vi "Actor Core.vi"(8 "error in (no error)":errorcluster, 11 "front_panel in":refnum<class "front_panel.lvclass">) -> (0 "error out":errorcluster, 3 "Actor out":refnum<class "Actor.lvclass">)   [LabVIEW 2015, in "front_panel.lvclass"]
doc: "(<B>Filename</B>: Actor Framework.lvlib:Actor.lvclass:Actor Core.vi)\n\nReceives messages to the actor, reacts to them, and initiates any error handling that may shut the actor down.\n\nDescendant classes may override this VI to append parallel tasks for the actor to complete while it handles messages. Overrides use the Call Parent Method node."
uses:
  front_panel.lvclass
  <vilib>/ActorFramework/Actor/Actor.lvclass
  stage_types.ctl
  experiment_types.ctl
  detector_types.ctl
  gui_subpanel_references.ctl
  ui_plot_references.ctl
  ui_elements.ctl
  front_panel.lvclass/front_panel.ctl
  panel_class/panel.lvclass/panel.ctl
  <vilib>/ActorFramework/Actor/Actor.lvclass/Actor.ctl
  <vilib>/ActorFramework/Message Enqueuer/Message Enqueuer.lvclass/Message Enqueuer.ctl
  front_panel Messages/replace_subpanel Msg/replace_subpanel Msg.lvclass/replace_subpanel Msg.ctl
  map_data.ctl
  <vilib>/Utility/miscctls.llb/LVOffsetAndMultiplierTypeDef.ctl
  <vilib>/ActorFramework/Message Enqueuer/Init from Existing Queue.vi
  <vilib>/ActorFramework/Message Enqueuer/Enqueue.vi
  <vilib>/ActorFramework/Message Priority Queue/Priority Enqueue.vi
  <vilib>/ActorFramework/Message Enqueuer/Message Enqueuer.lvclass
  <vilib>/ActorFramework/Stop Msg/Stop Msg.lvclass
  front_panel Messages/replace_subpanel Msg/replace_subpanel Msg.lvclass
  panel_class/panel.lvclass
panel:
  in  "stage1":T1
  in  "stage2":T1
  in  "experiment":T2
  in  "2.":T3
  in  "detector":T3
  in  "plots":T4(tab)
  in  "ch_4_color 2":u32(colorbox)=11141375 caption="6"
  in  "ch_3_color 2":u32(colorbox)=16768322 caption="5"
  out "Y Cursor":dbl
  out "X Cursor":dbl
  in  "ch_4_color":u32(colorbox)=3381759 caption="4"
  in  "ch_3_color":u32(colorbox)=6618880 caption="3"
  in  "ch_2_color":u32(colorbox)=16711680 caption="2"
  in  "ch_1_color":u32(colorbox)=13816530 caption="1"
  out "chart":cluster{dbl, dbl, dbl, dbl, dbl, dbl, dbl, dbl}(graph)
  out "graph":dbl[](graph)
  in  "load _map":bool
  in  "clear_maps":bool
  out "current":i32
  out "maps stored":i32
  in  "map_forward":bool
  in  "map_back":bool
  in  "keep_map":bool
  out "Y Cursor":dbl
  out "X Cursor":dbl
  out "map":dbl[][](graph)
  out "XY Graph":cluster{dbl[], dbl[]}[](graph)
  out "ch4":dbl
  out "ch3":dbl
  out "ch2":dbl
  out "ch1":dbl
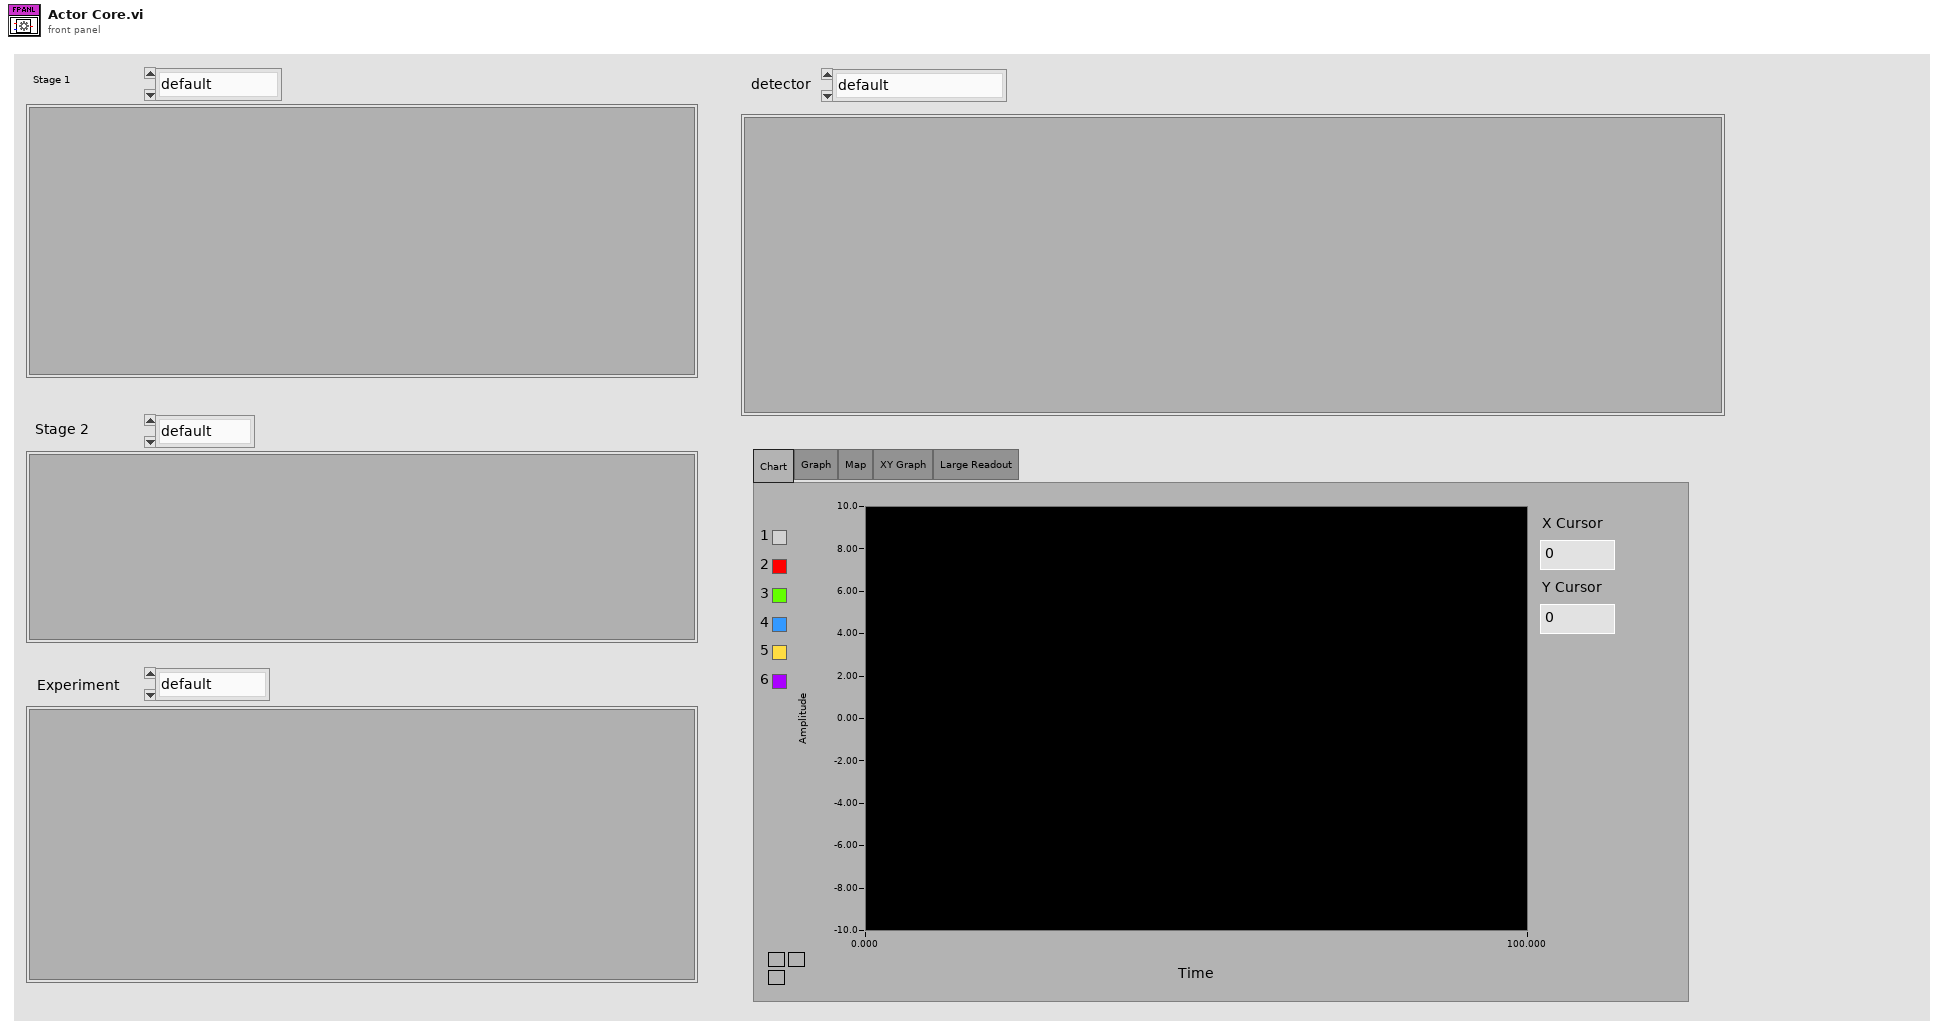
[diagram p1: front panel]
types:
  T1 = typedef "stage_types.ctl" = enum16{"default", "Newport XPS", "Aerotech Ensemble", "Galvos", "Throlabs Kinesis", "MCL XYZ Piezo"}
  T2 = typedef "experiment_types.ctl" = enum16{"default", "PCFS", "Scan", "2D Galvo Scan"}
  T3 = typedef "detector_types.ctl" = enum16{"default", "Hydraharp", "Picoharp", "Lightfield"}
  T4 = enum32{"Chart", "Graph", "Map", "XY Graph", "Large Readout"}
  T5 = typedef "ui_elements.ctl" = cluster{"map_xcursor":refnum<vi>, "map_ycursor":refnum<vi>}
  T6 = typedef "ui_plot_references.ctl" = cluster{"plots":refnum<vi>, "chart":refnum<vi>, "graph":refnum<vi>, "map":refnum<vi>, "XY Graph":refnum<vi>}
  T7 = typedef "gui_subpanel_references.ctl" = cluster{"Stage 1":refnum<vi>, "Stage 2":refnum<vi>, "Experiment":refnum<vi>, "Detector":refnum<vi>}
  T8 = typedef "ui_registered_events.ctl" = cluster{"update_xy_graph":refnum<event-registration>, "update_graph":refnum<event-registration>, "update_chart":refnum<event-registration>, "update_map":refnum<event-registration>, "event_loop_stop":refnum<event-registration>, "keep_map":refnum<event-registration>}
  T9 = typedef "map_data.ctl" = cluster{"data":dbl[][], "XScale.Ofst&Mult":T10, "YScale.Ofst&Mult":T10}
  T10 = typedef "LVOffsetAndMultiplierTypeDef.ctl" = cluster{"Offset":dbl, "Multiplier":dbl}
  T11 = typedef "LVPoint32TypeDef.ctl" = cluster{"Horizontal":i32, "Vertical":i32}
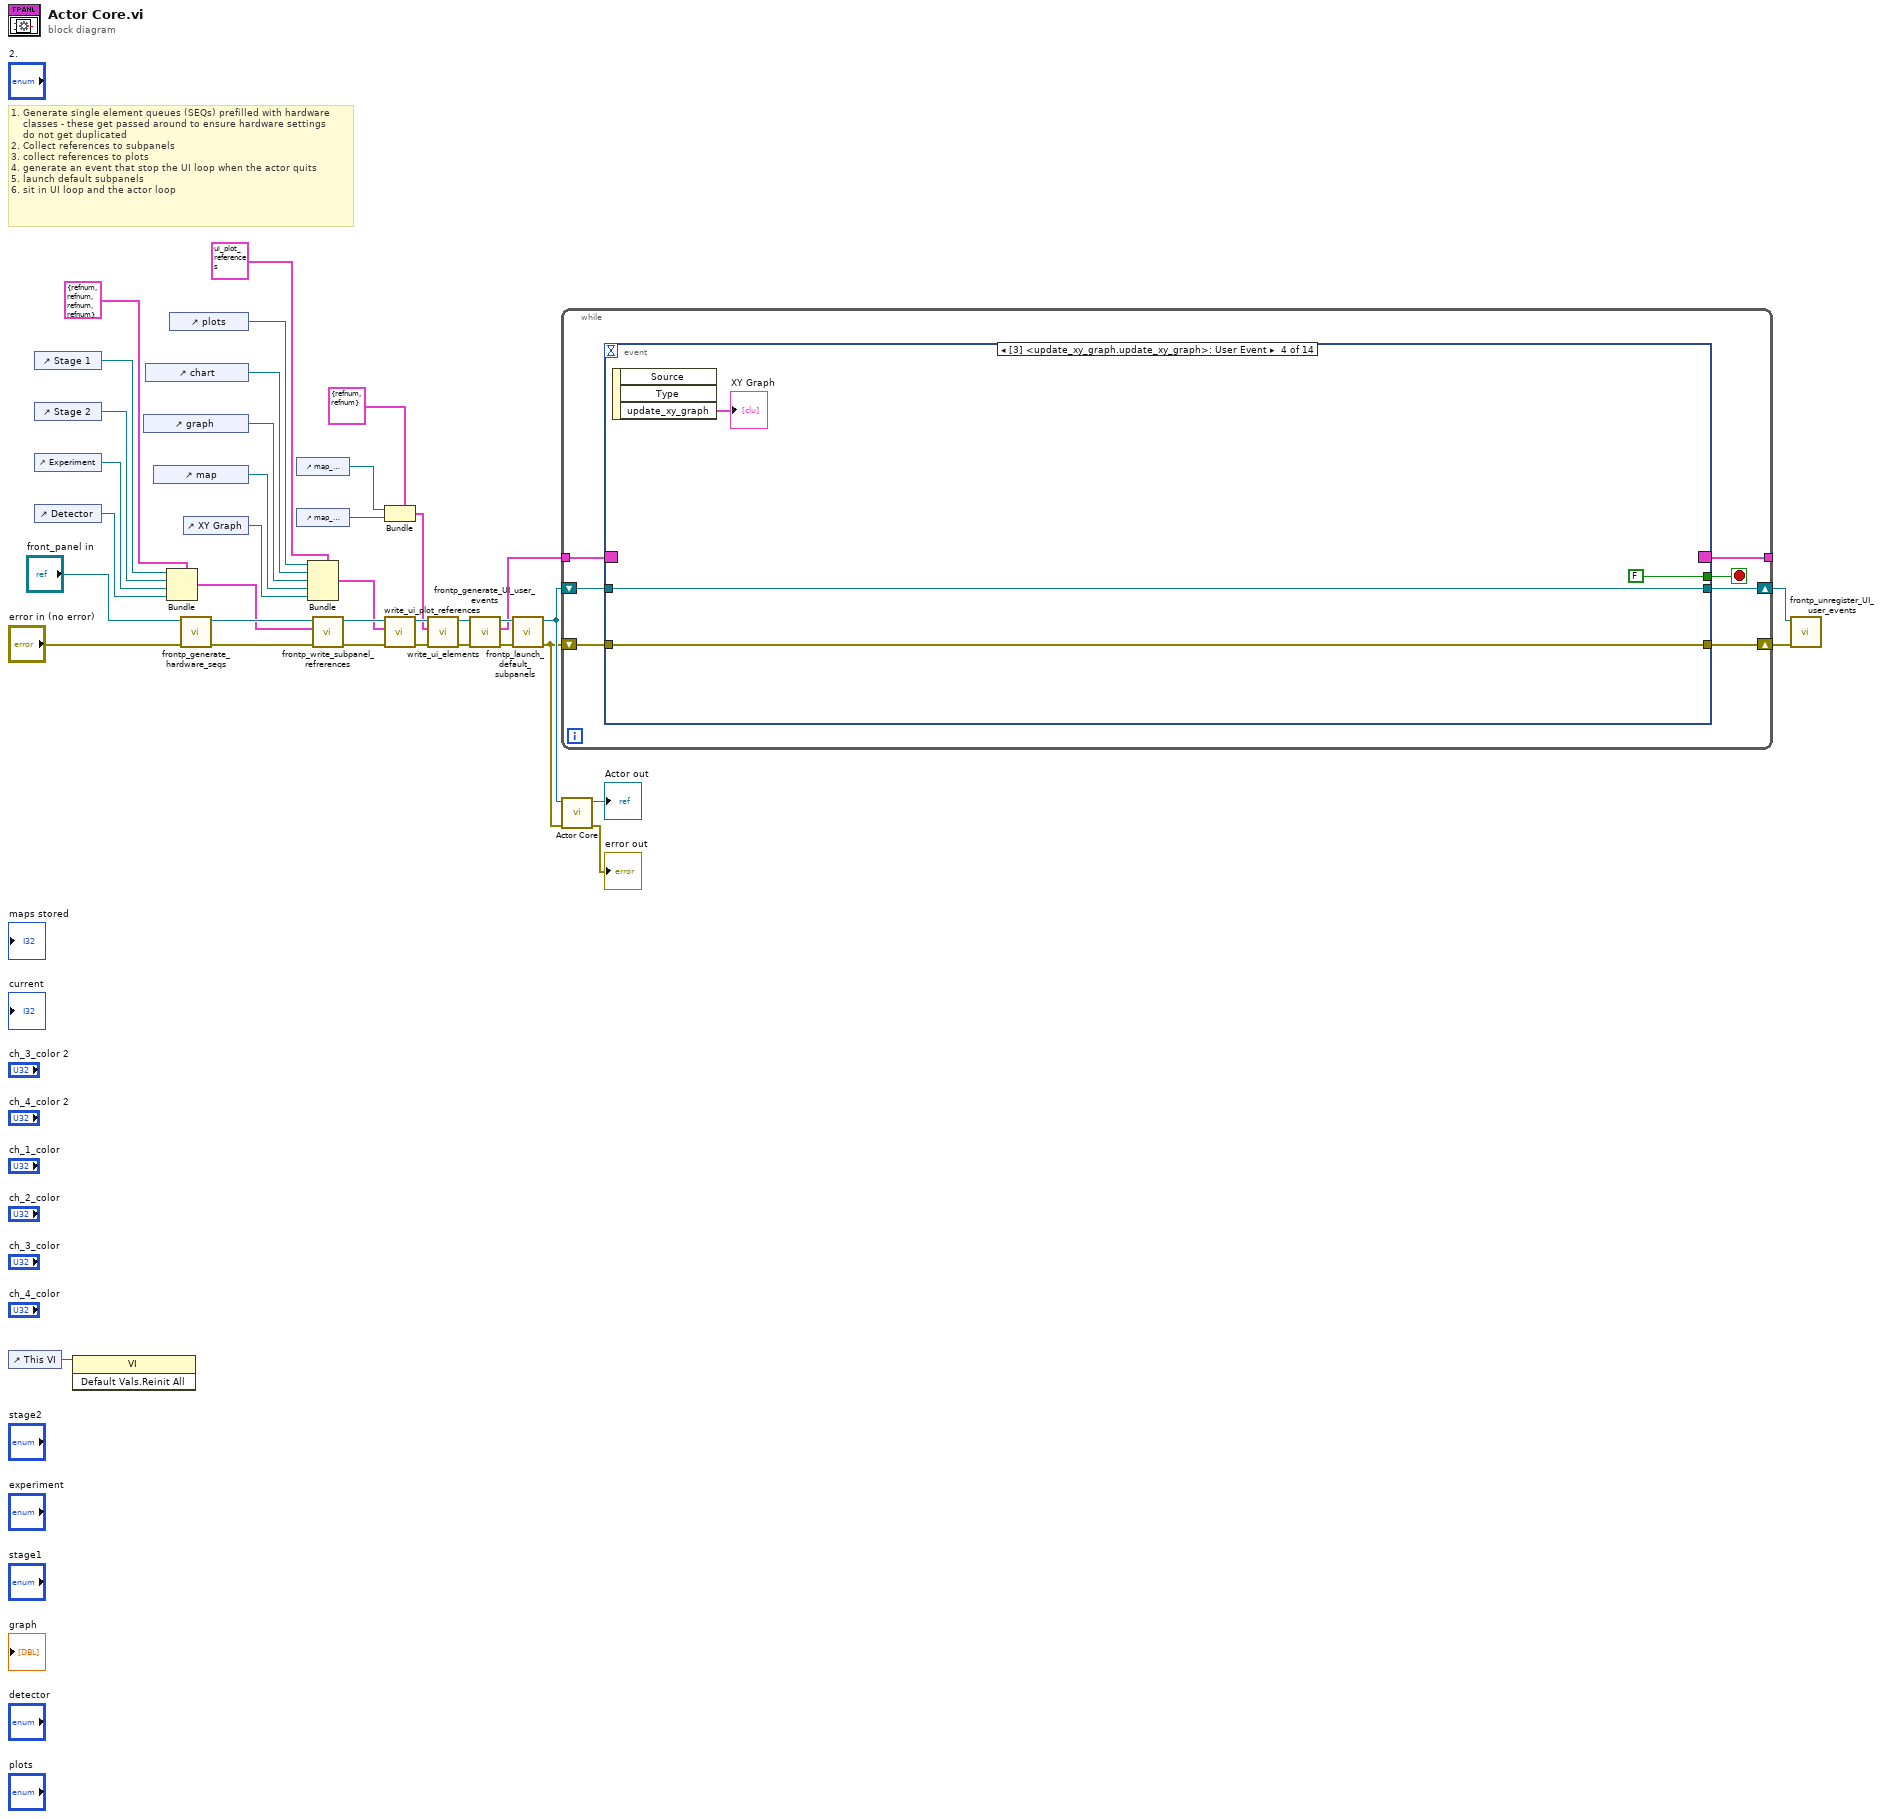
[diagram p0: block diagram]
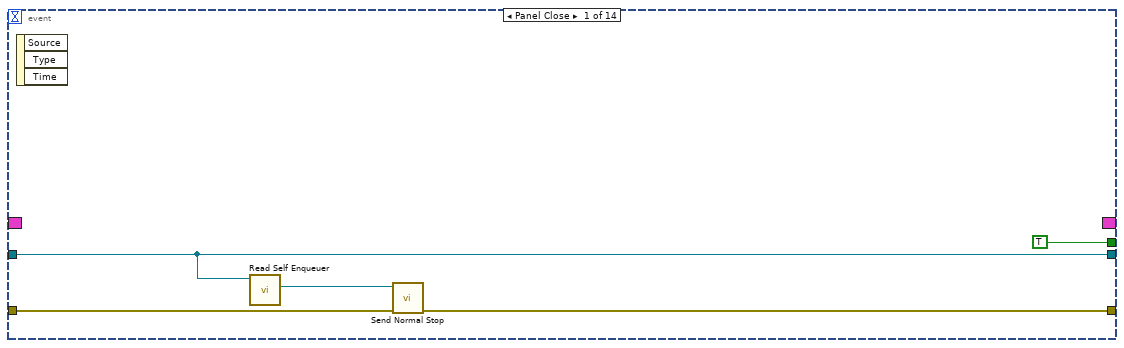
[diagram p2: hidden frame]
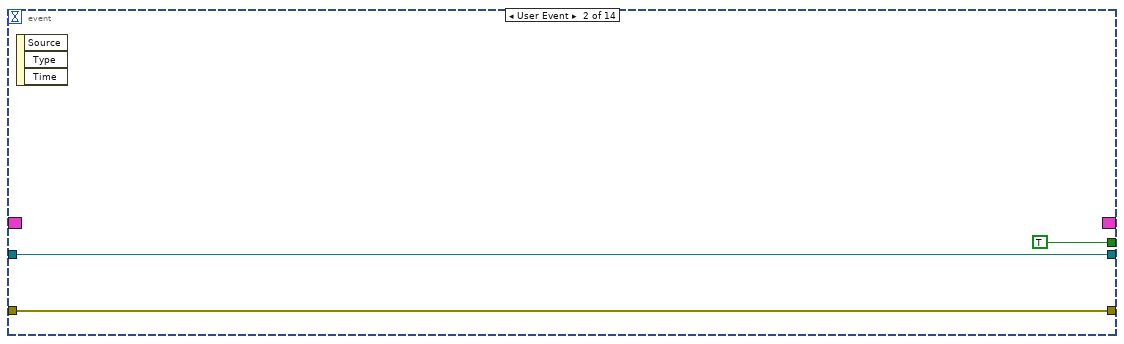
[diagram p3: hidden frame]
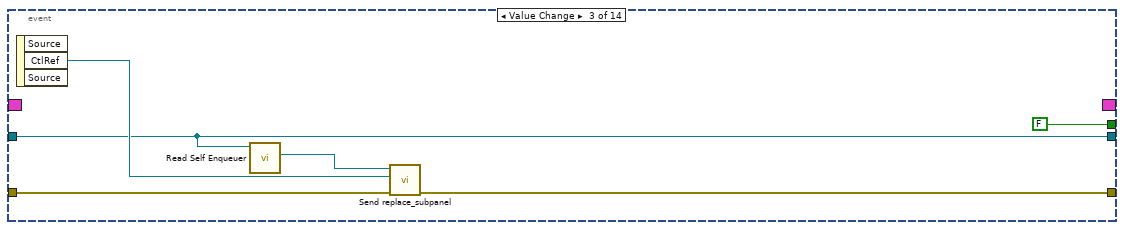
[diagram p4: hidden frame]
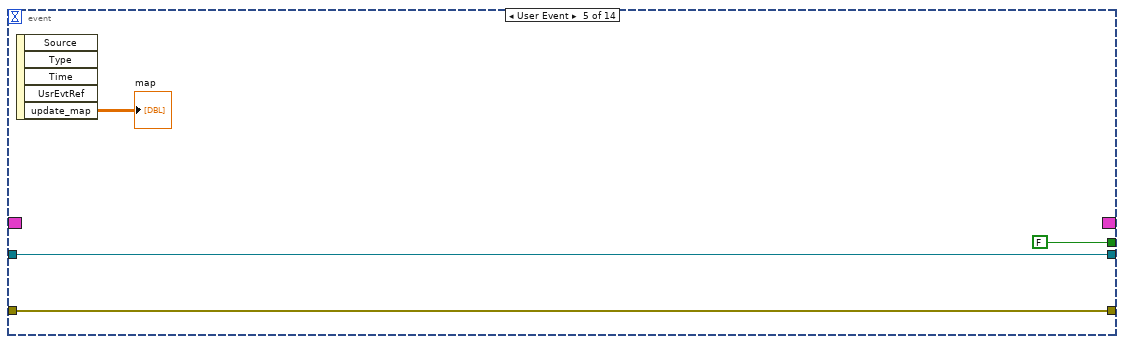
[diagram p5: hidden frame]
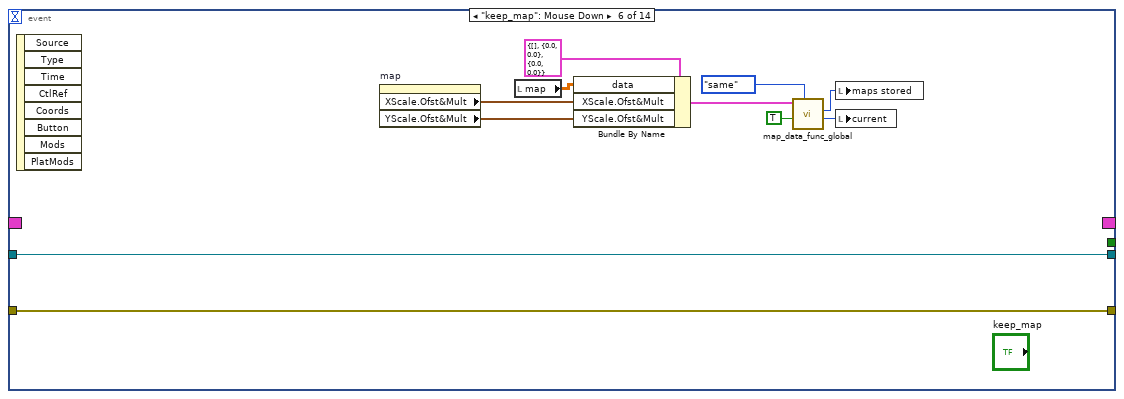
[diagram p6: hidden frame]
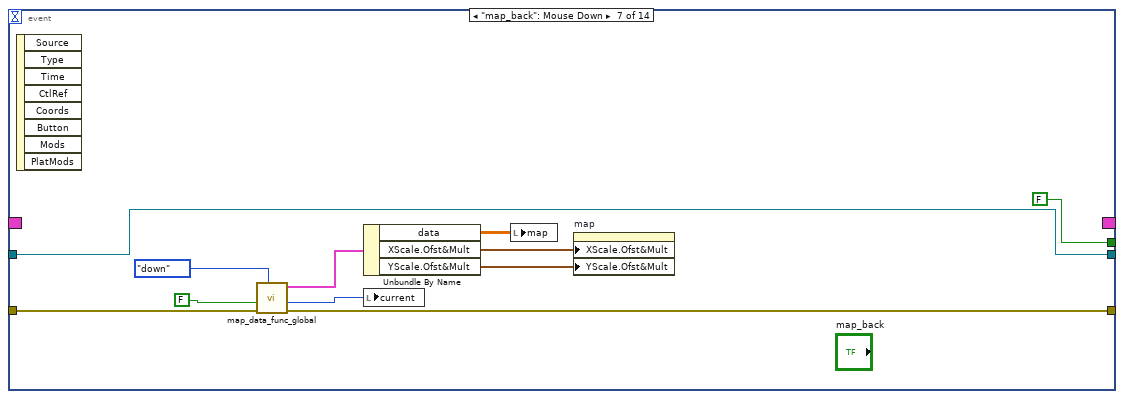
[diagram p7: hidden frame]
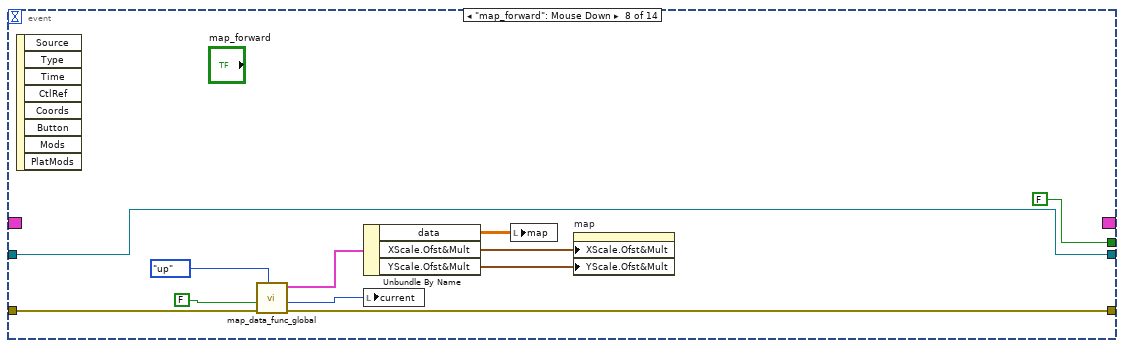
[diagram p8: hidden frame]
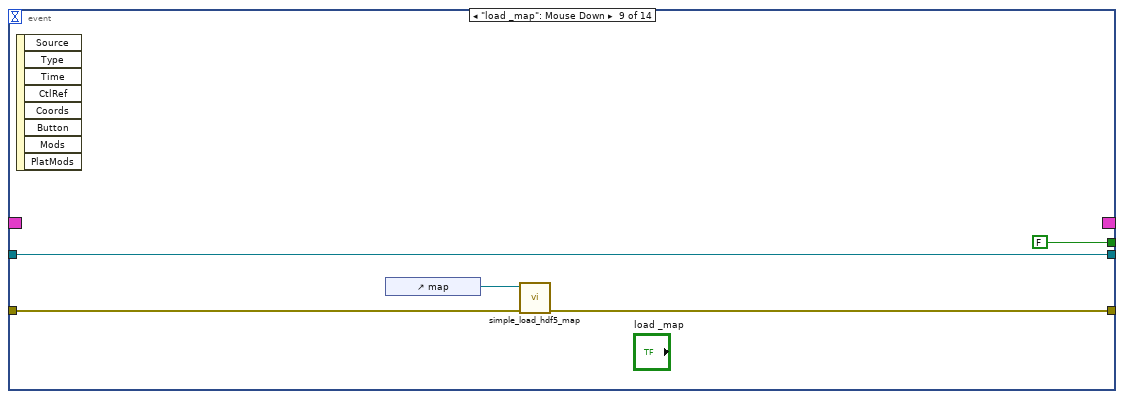
[diagram p9: hidden frame]
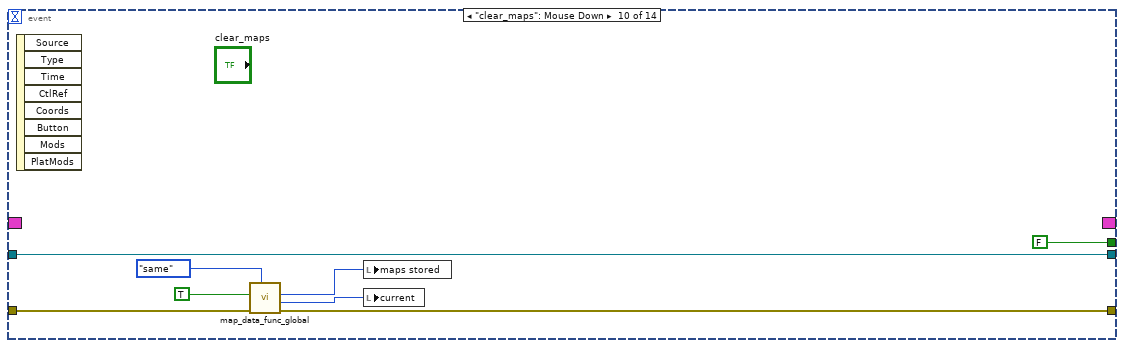
[diagram p10: hidden frame]
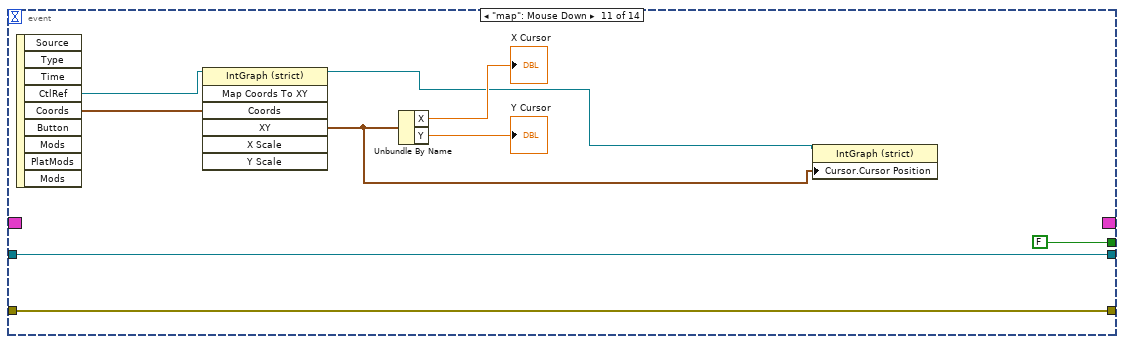
[diagram p11: hidden frame]
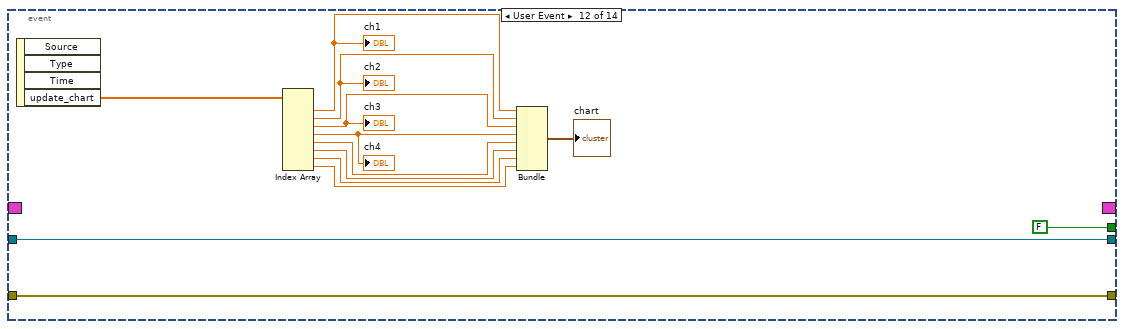
[diagram p12: hidden frame]
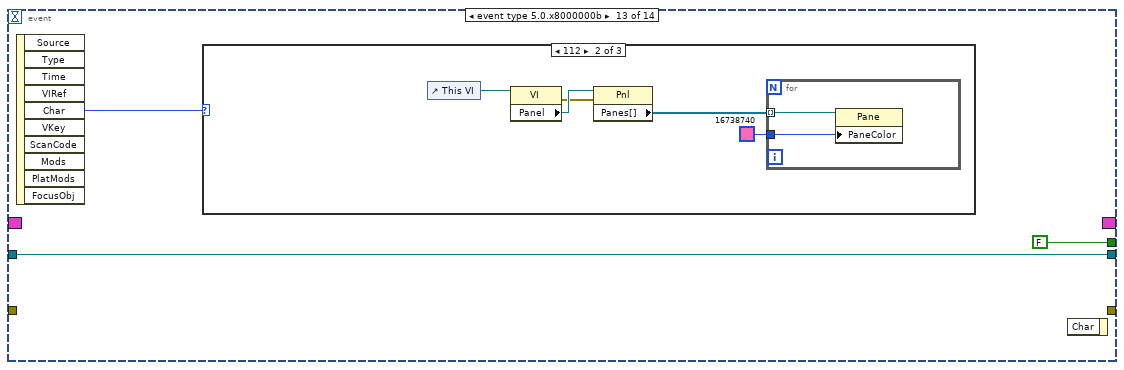
[diagram p13: hidden frame]
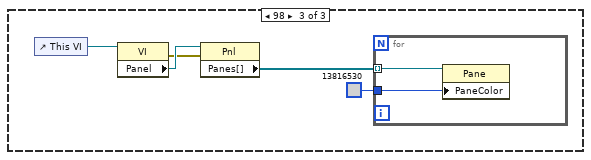
[diagram p15: hidden frame]
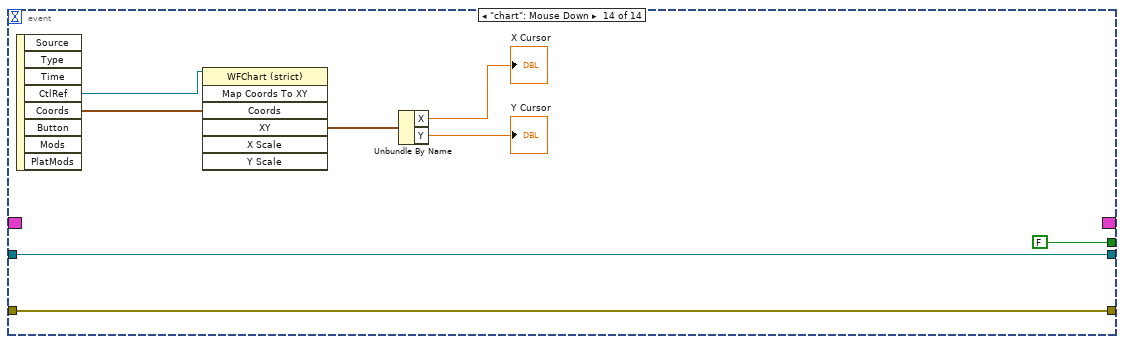
[diagram p16: hidden frame]
diagram:
  # "1. Generate single element queues (SEQs) prefilled with hardware\n    classes - these get passed around to ensure hardware settings\n    do not get duplicated\n2. Collect references to subpanels\n3. collect references to plots\n4. generate an event that stop the UI loop when the actor quits\n5. launch default subpanels\n6. sit in UI loop and the actor loop"
  n1 = control-ref of="This VI"() -> (w18:refnum<vi>)
  n2 = control-ref of="Stage 1"() -> (w37:refnum<vi>)
  n3 = control-ref of="Stage 2"() -> (w36:refnum<vi>)
  n4 = control-ref of="Experiment"() -> (w35:refnum<vi>)
  n5 = control-ref of="Detector"() -> (w34:refnum<vi>)
  n6 = invoke class="VI" method="Default Vals.Reinit All"(reference=w18) -> ()  [unwired: 2 in, 3 out]
  n7 = control-ref of="graph"() -> (w24:refnum<vi>)
  n8 = control-ref of="chart"() -> (w9:refnum<vi>)
  n9 = control-ref of="map"() -> (w23:refnum<vi>)
  n10 = Bundle(cluster=T7 {"Stage 1"=refnum, "Stage 2"=refnum, "Experiment"=refnum, "Detector"=refnum} ("output cluster"), "Stage 1"=w37, "Stage 2"=w36, "Experiment"=w35, "Detector"=w34) -> (w29:T7)
  n11 = control-ref of="plots"() -> (w25:refnum<vi>)
  n12 = call "frontp_generate_hardware_seqs.vi"("error in (no error)"="error in (no error)", "front_panel in"="front_panel in") -> ("error out"=w30:errorcluster, "front_panel out"=w31:refnum<class "front_panel.lvclass">)  [unwired: 8 in]
  n13 = control-ref of="XY Graph"() -> (w17:refnum<vi>)
  n14 = control-ref of="map_xcursor"() -> (w8:refnum<vi>)
  n15 = control-ref of="map_ycursor"() -> (w7:refnum<vi>)
  n16 = Bundle(cluster=T6 {"plots"=refnum, "chart"=refnum, "graph"=refnum, "map"=refnum, "XY Graph"=refnum} ("output cluster"), "plots"=w25, "chart"=w9, "graph"=w24, "map"=w23, "XY Graph"=w17) -> (w19:T6)
  n17 = call "frontp_write_subpanel_refrerences.vi"("error in (no error)"=w30, "GUI_subpanels"=w29, "front_panel in"=w31) -> ("error out"=w20:errorcluster, "front_panel out"=w21:refnum<class "front_panel.lvclass">)  [unwired: 7 in]
  n18 = Bundle(cluster=T5 {"map_xcursor"=refnum, "map_ycursor"=refnum} ("output cluster"), "map_xcursor"=w8, "map_ycursor"=w7) -> (w2:T5)
  n19 = call "write_ui_plot_references.vi"("error in (no error)"=w20, "plot_references"=w19, "panel in"=w21) -> ("error out"=w6:errorcluster, "panel out"=w5:refnum<class "front_panel.lvclass">)  [unwired: 7 in]
  n20 = call "write_ui_elements.vi"("error in (no error)"=w6, "ui_elements"=w2, "panel in"=w5) -> ("error out"=w3:errorcluster, "panel out"=w4:refnum<class "front_panel.lvclass">)  [unwired: 7 in]
  n21 = call "frontp_generate_UI_user_events.vi"("error in (no error)"=w3, "front_panel in"=w4) -> ("error out"=w11:errorcluster, "registred_events"=w15:T8, "front_panel out"=w16:refnum<class "front_panel.lvclass">)  [unwired: 7 in]
  n22 = call "frontp_launch_default_subpanels.vi"("error in (no error)"=w11, "front_panel in"=w16) -> ("error out"=w10:errorcluster, "front_panel out"=w13:refnum<class "front_panel.lvclass">)  [unwired: 8 in]
  n23 = while {
    shift-right: [w41] -> w14
    shift-left: w10 -> [w42]
    tunnel: [w43] -> _
    tunnel: w15 -> [w40]
    shift-right: [w38] -> w12
    shift-left: w13 -> [w39]
    stop <- w44 stop-if-true
    n24 = event shown="[3] <update_xy_graph.update_xy_graph>: User Event" {
      selector: w40 -> [_ _ _ _ _ _ _ _ _ _ _ _ _ _]
      dyn-events: [_ _ _ _ _ _ _ _ _ _ _ _ _ _] -> w43
      timeout: _ -> [_ _ _ _ _ _ _ _ _ _ _ _ _ _]
      tunnel: [TRUE TRUE FALSE FALSE FALSE _ FALSE FALSE FALSE FALSE FALSE FALSE FALSE FALSE] -> w44
      tunnel: w42 -> [w47 w51 w57 w59 w65 w77 w80 w95 w102 w110 w119 w131 _ w153]
      tunnel: [w48 w51 w54 w59 w65 w77 w79 w94 w101 w106 w119 w131 _ w153] -> w41
      tunnel: w39 -> [w45 w50 w53 w61 w66 w76 w88 w99 w104 w112 w121 w132 w136 w154]
      tunnel: [w45 w50 w53 w61 w66 w76 w88 w99 w104 w112 w121 w132 w136 w154] -> w38
      event Panel Close {
        n25 = event-data() -> ()  [unwired: 1 in, 3 out]
        n26 = call <vilib>:"Read Self Enqueuer.vi"("Actor"=w45) -> ("Self Enqueuer"=w46:refnum<class "Message Enqueuer.lvclass">)  [unwired: 10 in]
        n27 = call <vilib>:"Send Normal Stop.vi"("error in (no error)"=w47, "Message Enqueuer"=w46) -> ("error out"=w48:errorcluster)  [unwired: 9 in]
      }
      event User Event {
        n28 = event-data() -> ()  [unwired: 1 in, 3 out]
      }
      event Value Change {
        n29 = event-data() -> ("CtlRef"=w56:refnum<vi>)  [unwired: 1 in, 2 out]
        n30 = call <vilib>:"Read Self Enqueuer.vi"("Actor"=w53) -> ("Self Enqueuer"=w55:refnum<class "Message Enqueuer.lvclass">)  [unwired: 10 in]
        n31 = call "Send replace_subpanel.vi"("error in (no error)"=w57, "changed_subpanel"=w56, "Message Enqueuer"=w55) -> ("error out"=w54:errorcluster)  [unwired: 7 in, 1 out]
      }
      event User Event {
        n32 = event-data() -> ("update_xy_graph"=→"XY Graph":cluster{dbl[], dbl[]}[])  [unwired: 1 in, 2 out]
      }
      event User Event {
        n33 = event-data() -> ("update_map"=→"map":dbl[][])  [unwired: 1 in, 4 out]
      }
      event "keep_map": Mouse Down {
        n34 = event-data() -> ()  [unwired: 1 in, 8 out]
        n35 = property on="map" class="IntGraph (strict)"() -> ("XScale.Ofst&Mult"=w74:T10, "YScale.Ofst&Mult"=w73:T10)  [unwired: 2 in, 2 out]
        n36 = local read "map"() -> (w75:dbl[][])
        n37 = Bundle By Name(cluster=T9 {"data"=[], "XScale.Ofst&Mult"={"Offset"=0.0, "Multiplier"=0.0}, "YScale.Ofst&Mult"={"Offset"=0.0, "Multiplier"=0.0}} ("new element/subarray"), "data"=w75, "XScale.Ofst&Mult"=w74, "YScale.Ofst&Mult"=w73) -> (w71:T9)
        n38 = call "map_data_func_global.vi"("map_select"=enum16{"up", "down", "same"}."same", "write_map"=TRUE, "new_map"=w71) -> ("current_map"=w67:i32, "maps_stored"=w68:i32)  [unwired: 5 in, 2 out]
        n39 = local write "maps stored"(w68) -> ()
        n40 = local write "current"(w67) -> ()
      }
      event "map_back": Mouse Down {
        n41 = event-data() -> ()  [unwired: 1 in, 8 out]
        n42 = call "map_data_func_global.vi"("map_select"=enum16{"up", "down", "same"}."down", "error in (no error)"=w80, "write_map"=FALSE) -> ("error out"=w79:errorcluster, "current_map"=w78:i32, "map_out"=w84:T9)  [unwired: 5 in, 1 out]
        n43 = Unbundle By Name(w84) -> ("data"=w83:dbl[][], "XScale.Ofst&Mult"=w82:T10, "YScale.Ofst&Mult"=w81:T10)
        n44 = local write "current"(w78) -> ()
        n45 = local write "map"(w83) -> ()
        n46 = property on="map" class="IntGraph (strict)"("XScale.Ofst&Mult"=w82, "YScale.Ofst&Mult"=w81) -> ()  [unwired: 2 in, 2 out]
      }
      event "map_forward": Mouse Down {
        n47 = event-data() -> ()  [unwired: 1 in, 8 out]
        n48 = call "map_data_func_global.vi"("map_select"=enum16{"up", "down", "same"}."up", "error in (no error)"=w95, "write_map"=FALSE) -> ("error out"=w94:errorcluster, "current_map"=w89:i32, "map_out"=w93:T9)  [unwired: 5 in, 1 out]
        n49 = Unbundle By Name(w93) -> ("data"=w92:dbl[][], "XScale.Ofst&Mult"=w91:T10, "YScale.Ofst&Mult"=w90:T10)
        n50 = local write "current"(w89) -> ()
        n51 = local write "map"(w92) -> ()
        n52 = property on="map" class="IntGraph (strict)"("XScale.Ofst&Mult"=w91, "YScale.Ofst&Mult"=w90) -> ()  [unwired: 2 in, 2 out]
      }
      event "load _map": Mouse Down {
        n53 = event-data() -> ()  [unwired: 1 in, 8 out]
        n54 = control-ref of="map"() -> (w100:refnum<vi>)
        n55 = call "simple_load_hdf5_map.vi"("error in (no error)"=w102, "IntensityGraph in"=w100) -> ("error out"=w101:errorcluster)  [unwired: 9 in]
      }
      event "clear_maps": Mouse Down {
        n56 = event-data() -> ()  [unwired: 1 in, 8 out]
        n57 = call "map_data_func_global.vi"("map_select"=enum16{"up", "down", "same"}."same", "error in (no error)"=w110, "clear_map_array"=TRUE) -> ("error out"=w106:errorcluster, "current_map"=w107:i32, "maps_stored"=w108:i32)  [unwired: 5 in, 1 out]
        n58 = local write "maps stored"(w108) -> ()
        n59 = local write "current"(w107) -> ()
      }
      event "map": Mouse Down {
        n60 = event-data() -> ("CtlRef"=w115:refnum<vi>, "Coords"=w116:T11)  [unwired: 1 in, 7 out]
        n61 = invoke class="IntGraph (strict)" method="Map Coords To XY"(reference=w115, "Coords"=w116) -> (reference out=w113:refnum<vi>, "XY"=w114:cluster{"X":dbl, "Y":dbl})  [unwired: 5 in, 5 out]
        n62 = Unbundle By Name(w114) -> ("X"=→"X Cursor":dbl, "Y"=→"Y Cursor":dbl)
        n63 = property class="IntGraph (strict)"(reference=w113, "Cursor.Cursor Position"=w114) -> ()  [unwired: 1 in, 2 out]
      }
      event User Event {
        n64 = event-data() -> ("update_chart"=w134:dbl[])  [unwired: 1 in, 3 out]
        n65 = Index Array(array=w134) -> (element #1=w133:dbl, element #2=w129:dbl, element #3=w128:dbl, element #4=w127:dbl, element #5=w125:dbl, element #6=w124:dbl, element #7=w123:dbl, element #8=w122:dbl)  [unwired: 8 in]
        "ch1" <- w133
        "ch2" <- w129
        "ch3" <- w128
        "ch4" <- w127
        n66 = Bundle(w133, w129, w128, w127, w125, w124, w123, w122) -> (→"chart":cluster{dbl, dbl, dbl, dbl, dbl, dbl, dbl, dbl})  [unwired: 1 in]
      }
      event event type 5.0.x8000000b {
        n67 = event-data() -> ("Char"=w135:i16)  [unwired: 1 in, 9 out]
        n68 = case shown="112" w135 {
          frame Default {
          }
          frame 112 {
            n69 = control-ref of="This VI"() -> (w142:refnum<vi>)
            n70 = property class="VI"(reference=w142) -> (error out=w140:errorcluster, "Panel"=w141:refnum<vi>)  [unwired: 1 in, 1 out]
            n71 = property class="Pnl"(reference=w141, error in=w140) -> ("Panes[]"=w139:refnum<vi>[])  [unwired: 2 out]
            n72 = for {
              tunnel: w139 -> [w144] mode=indexing
              tunnel: u32 16738740 -> [w143]
              n73 = property class="Pane"(reference=w144, "PaneColor"=w143) -> ()  [unwired: 1 in, 2 out]
            }
          }
          frame 98 {
            n74 = control-ref of="This VI"() -> (w149:refnum<vi>)
            n75 = property class="VI"(reference=w149) -> (error out=w147:errorcluster, "Panel"=w148:refnum<vi>)  [unwired: 1 in, 1 out]
            n76 = property class="Pnl"(reference=w148, error in=w147) -> ("Panes[]"=w146:refnum<vi>[])  [unwired: 2 out]
            n77 = for {
              tunnel: w146 -> [w151] mode=indexing
              tunnel: u32 13816530 -> [w150]
              n78 = property class="Pane"(reference=w151, "PaneColor"=w150) -> ()  [unwired: 1 in, 2 out]
            }
          }
        }
        n79 = event-data() -> ()  [unwired: 2 in, 1 out]
      }
      event "chart": Mouse Down {
        n80 = event-data() -> ("CtlRef"=w159:refnum<vi>, "Coords"=w158:T11)  [unwired: 1 in, 6 out]
        n81 = invoke class="WFChart (strict)" method="Map Coords To XY"(reference=w159, "Coords"=w158) -> ("XY"=w157:cluster{"X":dbl, "Y":dbl})  [unwired: 5 in, 6 out]
        n82 = Unbundle By Name(w157) -> ("X"=→"X Cursor":dbl, "Y"=→"Y Cursor":dbl)
      }
    }
  }
  n83 = call-parent "Actor Core.vi"("error in"=w10, "Actor in"=w13) -> ("error out"=→"error out":errorcluster, "Actor out"=→"Actor out":refnum<class "Actor.lvclass">)  [unwired: 8 in]
  n84 = call "frontp_unregister_UI_user_events.vi"("error in (no error)"=w14, "front_panel in"=w12) -> ()  [unwired: 8 in, 2 out]
